vi "Wait for Life Cycle State.vi"(8 "error in (no error)":errorcluster, 9 "timeout in ms (-1)":i32=-1, 10 "Lifecycle State":T1, 11 "Process In":refnum<class "Debug View.lvclass">) -> (0 "error out":errorcluster, 1 "timed out?":bool, 3 "Process Out":refnum<class "Debug View.lvclass">)   [LabVIEW 2020]
doc: "Wait for the process to enter the specified life cycle state."
uses:
  Debug View.lvclass
  Lifecycle State.ctl
  Debug View.lvclass/Debug View.ctl
  <vilib>/Utility/error.llb/Clear Errors.vi
  <vilib>/Utility/error.llb/Error Cluster From Error Code.vi
  <vilib>/ErrorRing/Error Ring.xnode
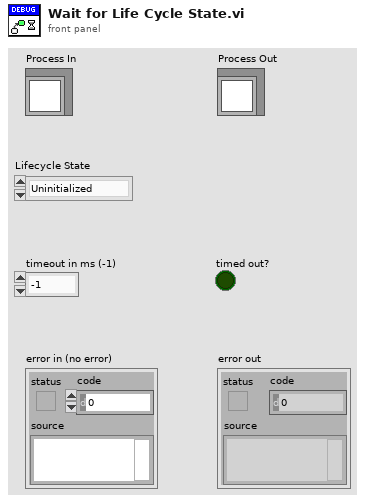
[diagram p1: front panel]
types:
  T1 = typedef "Lifecycle State.ctl" = enum16{"Uninitialized", "Initialized", "Started", "Running", "Stopped", "Finished"}
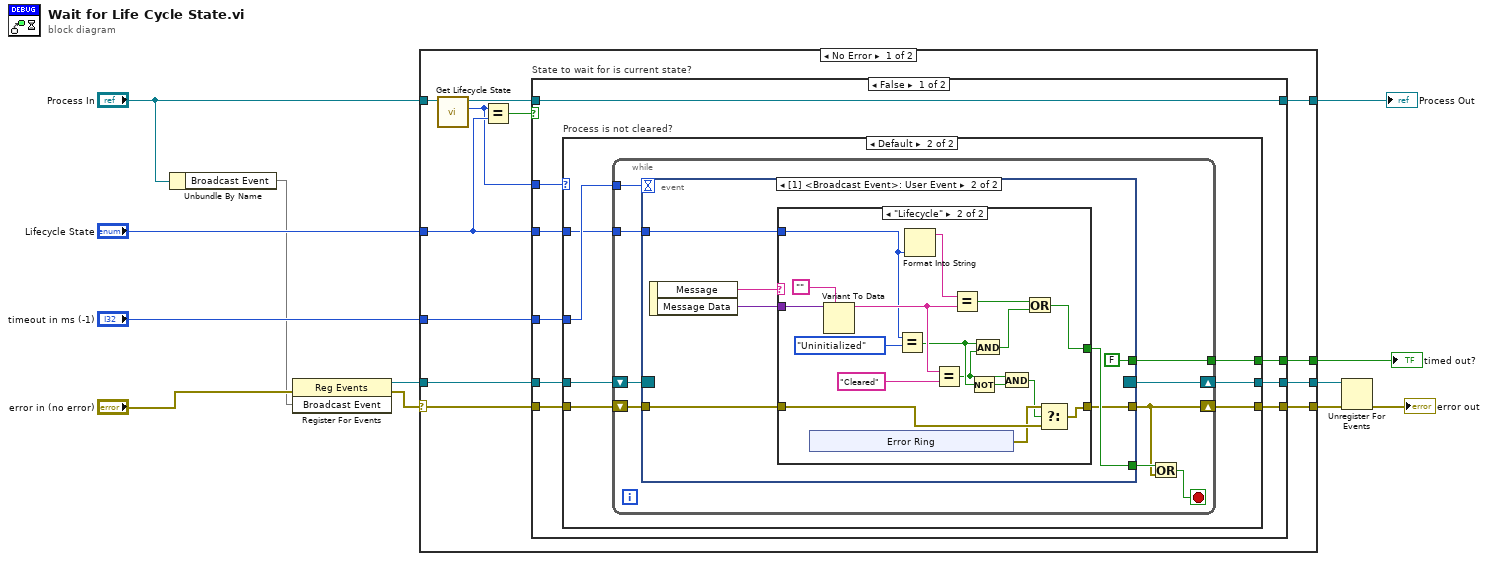
[diagram p0: block diagram]
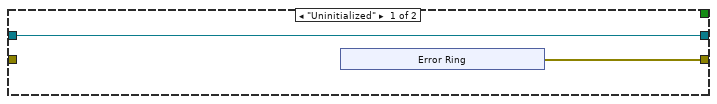
[diagram p2: hidden frame]
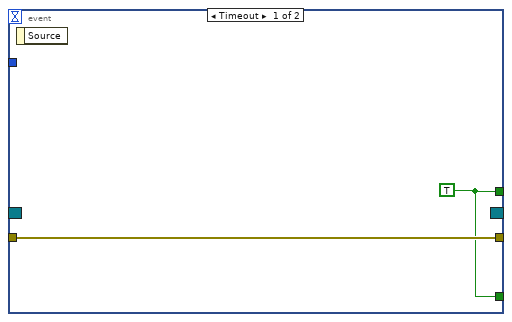
[diagram p3: hidden frame]
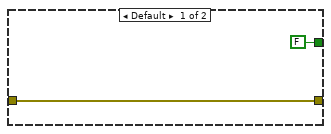
[diagram p4: hidden frame]
diagram:
  n1 = Unbundle By Name("Process In") -> ("Broadcast Event"=w5)
  n2 = register-events(error in="error in (no error)", w5) -> (reference out=w2:refnum<event-registration>, error out=w1:errorcluster)  [unwired: 1 in]
  n3 = case shown="No Error" w1 {
    selector: w1 -> [w16 w92]
    tunnel: "Process In" -> [w24 w91]
    tunnel: [w23 w91] -> w10
    tunnel: [w22 _] -> w9
    tunnel: "timeout in ms (-1)" -> [w21 _]
    tunnel: "Lifecycle State" -> [w14 _]
    tunnel: [w19 w92] -> w4
    tunnel: [w18 w93] -> w3
    tunnel: w2 -> [w17 w93]
    frame No Error {
      n4 = call "Get Lifecycle State.vi"("Process In"=w24) -> ("Lifecycle State"=w13:T1, "Process Out"=w20:refnum<class "Debug View.lvclass">)  [unwired: 7 in, 2 out]
      n5 = Equal?(x=w13, y=w14) -> (x = y?=w15:bool)
      n6 = case "State to wait for is current state?" shown="False" w15 {
        tunnel: [w27 w90] -> w23
        tunnel: w20 -> [w27 w90]
        tunnel: [w31 _] -> w22
        tunnel: [w28 w89] -> w19
        tunnel: w16 -> [w29 w89]
        tunnel: [w30 w88] -> w18
        tunnel: w17 -> [w33 w88]
        tunnel: w21 -> [w32 _]
        tunnel: w14 -> [w26 _]
        tunnel: w13 -> [w25 _]
        frame False {
          n7 = case "Process is not cleared?" shown="Default" w25 {
            tunnel: w33 -> [w34 w46]
            tunnel: w32 -> [_ w45]
            tunnel: [_ w44] -> w31
            tunnel: [w34 w43] -> w30
            tunnel: w29 -> [_ w42]
            tunnel: [w35 w41] -> w28
            tunnel: w26 -> [_ w40]
            frame "Uninitialized" {
              n8 = xnode "Error Ring"() -> ("error out"=w35:errorcluster)
            }
            frame Default {
              n9 = while {
                tunnel: w45 -> [w54]
                tunnel: [w53] -> w44
                shift-right: [w52] -> w43
                shift-left: w46 -> [w55]
                shift-right: [w47] -> w41
                shift-left: w42 -> [w51]
                tunnel: w40 -> [w49]
                stop <- w48 stop-if-true
                n10 = event shown="[1] <Broadcast Event>: User Event" {
                  selector: w55 -> [_ _]
                  dyn-events: [_ _] -> w52
                  timeout: w54 -> [_ _]
                  tunnel: [w56 FALSE] -> w53
                  tunnel: w51 -> [w57 w59]
                  tunnel: [w57 w58] -> w47
                  tunnel: [w56 w61] -> w50
                  tunnel: w49 -> [_ w62]
                  event Timeout {
                    w56 = TRUE
                    n11 = event-data() -> ()  [unwired: 1 in, 1 out]
                  }
                  event User Event {
                    n12 = event-data() -> ("Message"=w64:string, "Message Data"=w63:variant)  [unwired: 1 in]
                    n13 = case shown="\"Lifecycle\"" w64 {
                      tunnel: w63 -> [_ w83]
                      tunnel: w62 -> [_ w78]
                      tunnel: [FALSE w76] -> w61
                      tunnel: w59 -> [w65 w75]
                      tunnel: [w65 w73] -> w58
                      frame Default {
                      }
                      frame "Lifecycle" {
                        n14 = xnode "Error Ring"() -> ("error out"=w74:errorcluster)
                        n15 = Variant To Data(type="", Variant=w83) -> (data=w79:string)  [unwired: 1 in, 1 out]
                        n16 = Equal?(x=w78, y=Lifecycle_State."Uninitialized" ("Lifecycle State")) -> (x = y?=w71:bool)
                        n17 = Format Into String(w78) -> (resulting string=w81:string)  [unwired: 3 in, 1 out]
                        n18 = Equal?(x=w79, y="Cleared") -> (x = y?=w69:bool)
                        n19 = Equal?(x=w81, y=w79) -> (x = y?=w77:bool)
                        n20 = Not(x=w71) -> (.not. x?=w70:bool)
                        n21 = And(x=w71, y=w69) -> (x .and. y?=w72:bool)
                        n22 = And(x=w69, y=w70) -> (x .and. y?=w68:bool)
                        n23 = Or(x=w77, y=w72) -> (x .or. y?=w76:bool)
                        n24 = Select(t=w74, s=w68, f=w75) -> (s? t:f=w73:errorcluster)
                      }
                    }
                  }
                }
                n25 = Or(x=w50, y=w47) -> (x .or. y?=w48:bool)
              }
            }
          }
        }
        frame True {
        }
      }
    }
    frame Error {
    }
  }
  "Process Out" <- w10
  "timed out?" <- w9
  n26 = Unregister For Events(event registration refnum=w3, error in=w4) -> (error out=→"error out":errorcluster)
